vi "setHeater.vi"(6 "Channel":i32, 8 "error in (no error)":errorcluster, 10 "Current (A)":dbl, 11 "Instrument.Cryostat in":refnum<class "Instrument.Cryostat.lvclass">) -> (0 "error out":errorcluster, 3 "Instrument.Cryostat out":refnum<class "Instrument.Cryostat.lvclass">)   [LabVIEW 2019, in "Instrument.Cryostat.lvclass"]
uses:
  Instrument.Cryostat.lvclass
  C:/Users/patrick/Documents/GitHub/Instrument-Framework/lvsrc/Framework/Instrument/Instrument.lvclass
  Typedefs/setHeater--cluster.ctl
  Typedefs/Cryostat.commands--enum.ctl
  Instrument/Instrument.lvclass
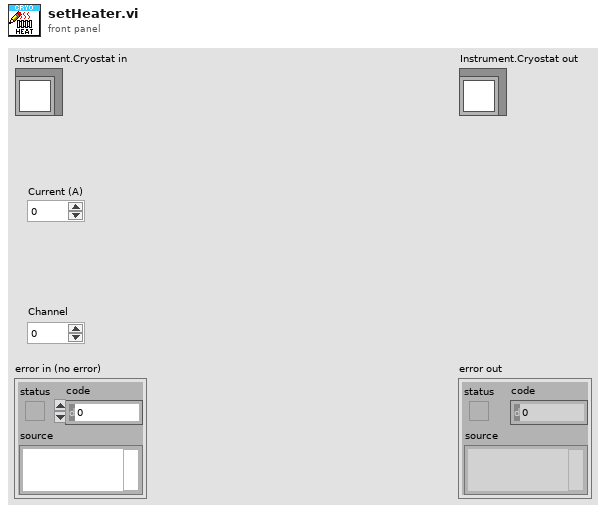
[diagram p1: front panel]
types:
  T1 = typedef "Instrument.Cryostat.lvclass/Cryostat.commands--enum.ctl" = enum16{"getLN2Level", "getLHeLevel", "getMagnet", "getMagnetVector", "setMagnet", "setMagnetVector", "getAngle", "setAngle", "getTemperature", "setTemperature", "getHeater", "setHeater", "getChamber", "setChamber", "getPressure"}
  T2 = typedef "Instrument.Cryostat.lvclass/setHeater--cluster.ctl" = cluster{"current":dbl, "channel":i32}
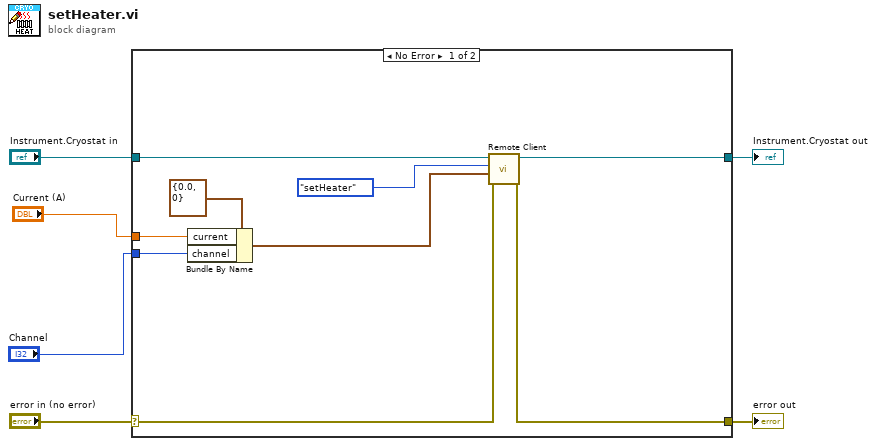
[diagram p0: block diagram]
diagram:
  n1 = case shown="No Error" "error in (no error)" {
    selector: "error in (no error)" -> [w8 w17]
    tunnel: [w11 w17] -> w5
    tunnel: [w12 w16] -> w3
    tunnel: "Instrument.Cryostat in" -> [w9 w16]
    tunnel: "Current (A)" -> [w15 _]
    tunnel: "Channel" -> [w14 _]
    frame No Error {
      n2 = Bundle By Name(cluster=T2 {"current"=0.0, "channel"=0} ("Set Temperature"), "current"=w15, "channel"=w14) -> (w7:T2)
      n3 = call "Remote Client.vi"("error in (no error)"=w8, "Data in"=w7, "Command in"=Cryostat.commands--enum."setHeater" ("commands"), "Instrument in"=w9) -> ("error out"=w11:errorcluster, "Instrument out"=w12:refnum<class "Instrument.Cryostat.lvclass">)  [unwired: 4 in, 2 out]
    }
    frame Error {
    }
  }
  "error out" <- w5
  "Instrument.Cryostat out" <- w3
